vi "Module Name--constant.vi"() -> (3 "Module Name":string)   [LabVIEW 2023, in "helloDqmhWorldModule.lvlib"]
doc: "Return the name of the module that owns this VI. \n_____\nBased on DQMH Project Template 7.0.0.1280."
uses:
  helloDqmhWorldModule.lvlib
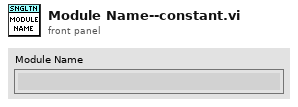
[diagram p1: front panel]
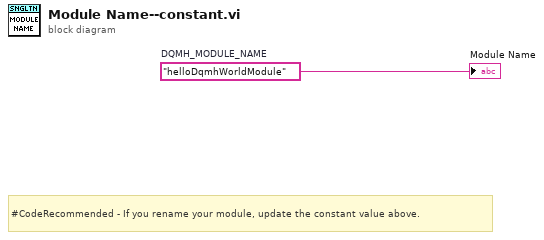
[diagram p0: block diagram]
diagram:
  w1 = "helloDqmhWorldModule"  # DQMH_MODULE_NAME
  # "#CodeRecommended - If you rename your module, update the constant value above."
  "Module Name" <- w1
